vi "PathPlanner_Trajectory_CalculateMaxVel.vi"(8 "Reversed":bool, 9 "MaxAccel":dbl, 10 "MaxVel":dbl, 11 "PathPlannerStates":T1[](array[typedef]) {"HolonomicRotation"."SIN" format="%13.4f"; "HolonomicRotation"."COS" format="%13.4f"; "HolonomicRotation"."VALUE" format="%13.4f"; "AngularVelocity"."SIN" format="%13.4f"; "AngularVelocity"."COS" format="%13.4f"; "AngularVelocity"."VALUE" format="%13.4f"; "TrajectoryState"."POSE"."ROTATION"."SIN" format="%13.4f"; "TrajectoryState"."POSE"."ROTATION"."COS" format="%13.4f"; "TrajectoryState"."POSE"."ROTATION"."VALUE" format="%13.4f"; "TrajectoryState"."POSE"."TRANSLATION"."Y" format="%14.3f"; "TrajectoryState"."POSE"."TRANSLATION"."X" format="%14.3f"; "AngularAcceleration"."SIN" format="%13.4f"; "AngularAcceleration"."COS" format="%13.4f"; "AngularAcceleration"."VALUE" format="%13.4f"}) -> (3 "outPathPlannerStates":T1[](array[typedef]) {"HolonomicRotation"."SIN" format="%13.4f"; "HolonomicRotation"."COS" format="%13.4f"; "HolonomicRotation"."VALUE" format="%13.4f"; "AngularVelocity"."SIN" format="%13.4f"; "AngularVelocity"."COS" format="%13.4f"; "AngularVelocity"."VALUE" format="%13.4f"; "TrajectoryState"."POSE"."ROTATION"."SIN" format="%13.4f"; "TrajectoryState"."POSE"."ROTATION"."COS" format="%13.4f"; "TrajectoryState"."POSE"."ROTATION"."VALUE" format="%13.4f"; "TrajectoryState"."POSE"."TRANSLATION"."Y" format="%14.3f"; "TrajectoryState"."POSE"."TRANSLATION"."X" format="%14.3f"; "AngularAcceleration"."SIN" format="%13.4f"; "AngularAcceleration"."COS" format="%13.4f"; "AngularAcceleration"."VALUE" format="%13.4f"})   [LabVIEW 2019, in "PathPlanner.lvlib"]
uses:
  PathPlanner.lvlib
  PathPlannerState.ctl
  <vilib>/Rock Robotics/WPI/ThirdParty/JAS_Junk/TrajLib/ROTATION2D.ctl
  <vilib>/Rock Robotics/WPI/ThirdParty/JAS_Junk/TrajLib/TRAJ_STATE.ctl
  <vilib>/Rock Robotics/WPI/ThirdParty/JAS_Junk/TrajLib/POSE2D.ctl
  <vilib>/Rock Robotics/WPI/ThirdParty/JAS_Junk/TrajLib/TRANSLATION2D.ctl
  <vilib>/Rock Robotics/WPI/ThirdParty/JAS_Junk/TrajLib/Trajectory_Library.lvlib
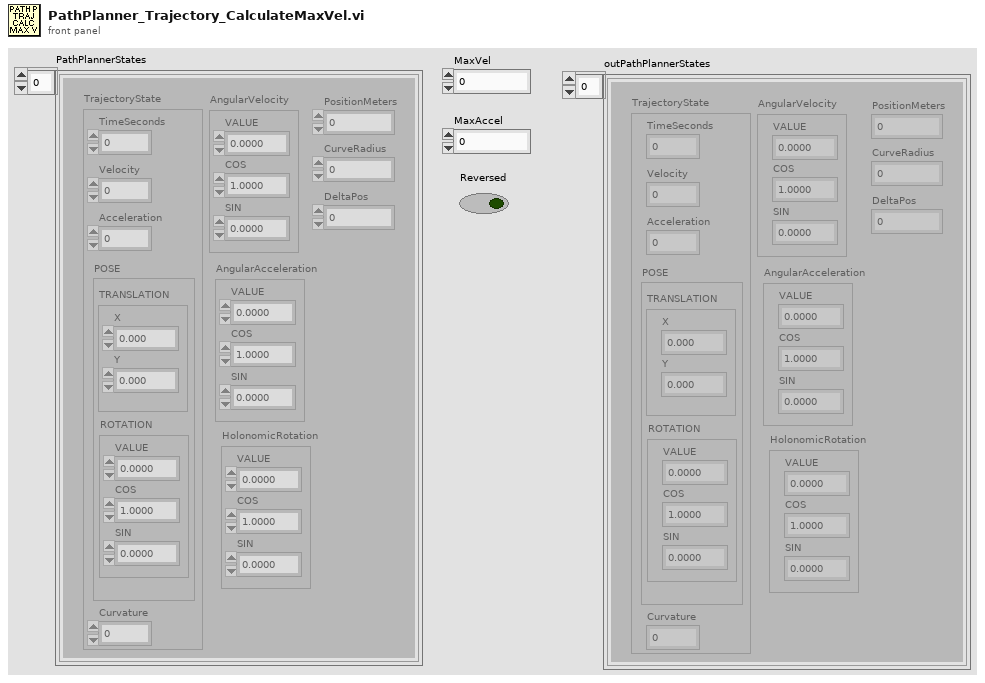
[diagram p1: front panel]
types:
  T1 = typedef "PathPlanner.lvlib/PathPlannerState.ctl" = cluster{"AngularAcceleration":T2, "PositionMeters":dbl, "TrajectoryState":T3, "AngularVelocity":T2, "HolonomicRotation":T2, "CurveRadius":dbl, "DeltaPos":dbl}
  T2 = typedef "Trajectory_Library.lvlib/ROTATION2D.ctl" = cluster{"VALUE":dbl, "COS":dbl, "SIN":dbl}
  T3 = typedef "Trajectory_Library.lvlib/TRAJ_STATE.ctl" = cluster{"TimeSeconds":dbl, "Velocity":dbl, "Acceleration":dbl, "POSE":T4, "Curvature":dbl}
  T4 = typedef "Trajectory_Library.lvlib/POSE2D.ctl" = cluster{"TRANSLATION":T5, "ROTATION":T2}
  T5 = typedef "Trajectory_Library.lvlib/TRANSLATION2D.ctl" = cluster{"X":dbl, "Y":dbl}
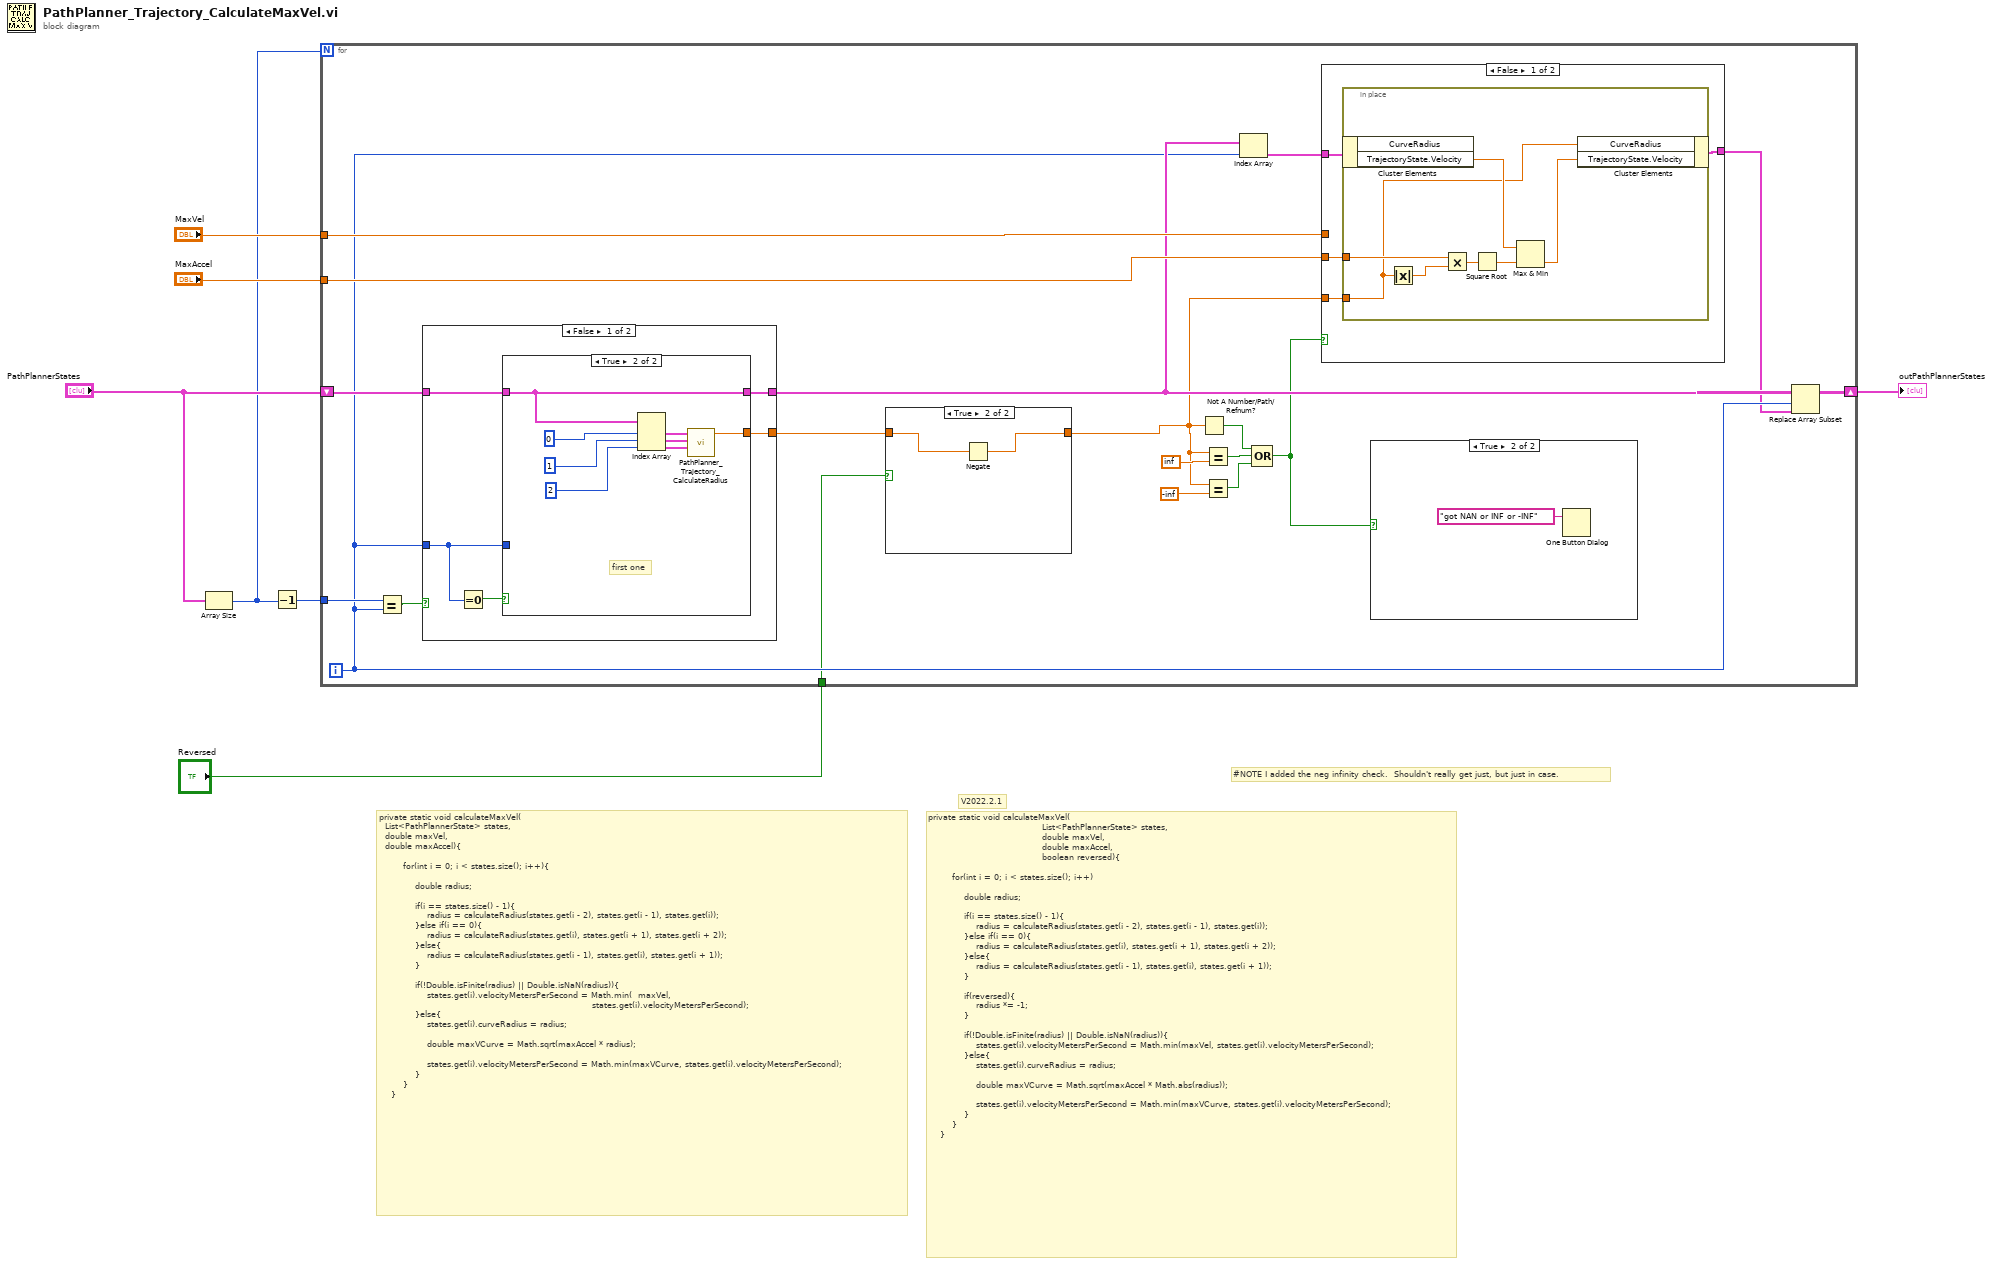
[diagram p0: block diagram]
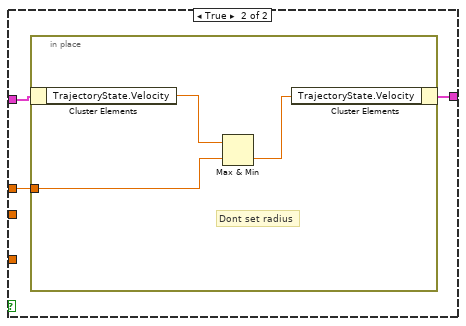
[diagram p4: hidden frame]
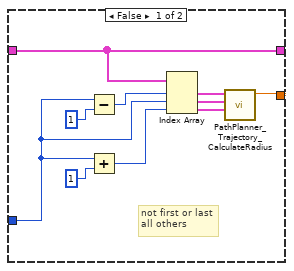
[diagram p5: hidden frame]
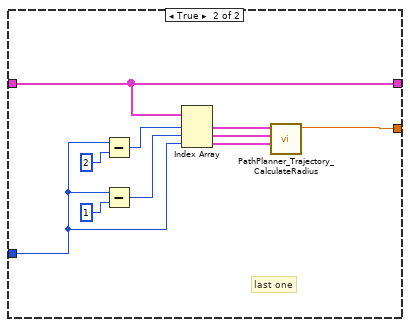
[diagram p6: hidden frame]
diagram:
  # "V2022.2.1"
  # "private static void calculateMaxVel(\n                                      List<PathPlannerState> states, \n                                      double maxVel, \n                                      double maxAccel, \n                                      boolean reversed){\n\n        for(int i = 0; i < states.size(); i++)\n\n            double radius;\n\n            if(i == states.size() - 1){\n                radius = calculateRadius(states.get(i - 2), states.get(i - 1), states.get(i));\n            }else if(i == 0){\n                radius = calculateRadius(states.get(i), states.get(i + 1), states.get(i + 2));\n            }else{\n                radius = calculateRadius(states.get(i - 1), states.get(i), states.get(i + 1));\n            }\n\n            if(reversed){\n                radius *= -1;\n            }\n\n            if(!Double.isFinite(radius) || Double.isNaN(radius)){\n                states.get(i).velocityMetersPerSecond = Math.min(maxVel, states.get(i).velocityMetersPerSecond);\n            }else{\n                states.get(i).curveRadius = radius;\n\n                double maxVCurve = Math.sqrt(maxAccel * Math.abs(radius));\n\n                states.get(i).velocityMetersPerSecond = Math.min(maxVCurve, states.get(i).velocityMetersPerSecond);\n            }\n        }\n    }"
  # "private static void calculateMaxVel(\n\t\tList<PathPlannerState> states, \n\t\tdouble maxVel, \n\t\tdouble maxAccel){\n\n        for(int i = 0; i < states.size(); i++){\n\n            double radius;\n\n            if(i == states.size() - 1){\n                radius = calculateRadius(states.get(i - 2), states.get(i - 1), states.get(i));\n            }else if(i == 0){\n                radius = calculateRadius(states.get(i), states.get(i + 1), states.get(i + 2));\n            }else{\n                radius = calculateRadius(states.get(i - 1), states.get(i), states.get(i + 1));\n            }\n\n            if(!Double.isFinite(radius) || Double.isNaN(radius)){\n                states.get(i).velocityMetersPerSecond = Math.min(  maxVel, \n\t\t\t\t                                                                   states.get(i).velocityMetersPerSecond);\n            }else{\n                states.get(i).curveRadius = radius;\n\n                double maxVCurve = Math.sqrt(maxAccel * radius);\n\n                states.get(i).velocityMetersPerSecond = Math.min(maxVCurve, states.get(i).velocityMetersPerSecond);\n            }\n        }\n    }"
  # "#NOTE I added the neg infinity check.  Shouldn't really get just, but just in case."
  n1 = Array Size(array="PathPlannerStates") -> (size(s)=w2:i32)
  n2 = Decrement(x=w2) -> (x-1=w7:i32)
  n3 = for {
    N: w2 -> [_]
    tunnel: w7 -> [w26]
    tunnel: "MaxVel" -> [w18]
    tunnel: "MaxAccel" -> [w17]
    shift-right: [w15] -> w3
    shift-left: "PathPlannerStates" -> [w24]
    tunnel: "Reversed" -> [w8]
    i -> [w13]
    n4 = Equal?(x=w26, y=w13) -> (x = y?=w25:bool)
    n5 = case shown="False" w25 {
      tunnel: w24 -> [w51 w71]
      tunnel: w13 -> [w49 w76]
      tunnel: [w50 w72] -> w10
      tunnel: [w48 w71] -> w14
      frame False {
        n6 = Equal To 0?(x=w49) -> (x = 0?=w52:bool)
        n7 = case shown="True" w52 {
          tunnel: w51 -> [w53 w63]
          tunnel: [w54 w64] -> w50
          tunnel: w49 -> [w56 _]
          tunnel: [w53 w63] -> w48
          frame False {
            # "not first or last\nall others"
            n8 = Subtract(x=w56, y=1) -> (x-y=w60:i32)
            n9 = Add(x=w56, y=1) -> (x+y=w55:i32)
            n10 = Index Array(array=w53, index #1=w60, index #2=w56, index #3=w55) -> (element #1=w59:T1, element #2=w58:T1, element #3=w57:T1)
            n11 = call "PathPlanner_Trajectory_CalculateRadius.vi"("S2"=w57, "S1"=w58, "S0"=w59) -> ("Radius"=w54:dbl)  [unwired: 8 in]
          }
          frame True {
            # "first one"
            n12 = Index Array(array=w63, index #1=0 ("y"), index #2=1 ("y"), index #3=2 ("y")) -> (element #1=w70:T1, element #2=w69:T1, element #3=w68:T1)
            n13 = call "PathPlanner_Trajectory_CalculateRadius.vi"("S2"=w68, "S1"=w69, "S0"=w70) -> ("Radius"=w64:dbl)  [unwired: 8 in]
          }
        }
      }
      frame True {
        # "last one"
        n14 = Subtract(x=w76, y=2) -> (x-y=w78:i32)
        n15 = Subtract(x=w76, y=1) -> (x-y=w77:i32)
        n16 = Index Array(array=w71, index #1=w78, index #2=w77, index #3=w76) -> (element #1=w75:T1, element #2=w74:T1, element #3=w73:T1)
        n17 = call "PathPlanner_Trajectory_CalculateRadius.vi"("S2"=w73, "S1"=w74, "S0"=w75) -> ("Radius"=w72:dbl)  [unwired: 8 in]
      }
    }
    n18 = case shown="True" w8 {
      tunnel: w10 -> [w27 w29]
      tunnel: [w27 w28] -> w9
      frame False {
      }
      frame True {
        n19 = Negate(x=w29) -> (-x=w28:dbl)
      }
    }
    n20 = Not A Number/Path/Refnum?(number/path/refnum=w9) -> (NaN/Path/Refnum?=w21:bool)
    n21 = Equal?(x=w9, y=inf) -> (x = y?=w20:bool)
    n22 = Equal?(x=w9, y=-inf) -> (x = y?=w19:bool)
    n23 = Index Array(array=w14, index=w13) -> (element=w16:T1)
    n24 = Compound Arithmetic op=OR(w21, w20, w19) -> (w11:bool)
    n25 = case shown="False" w11 {
      tunnel: [w34 w44] -> w12
      tunnel: w18 -> [_ w43]
      tunnel: w9 -> [w33 _]
      tunnel: w17 -> [w32 _]
      tunnel: w16 -> [w31 w42]
      frame False {
        n26 = in-place {
          in-place-border: w33 -> [w36]
          in-place-border: w32 -> [w41]
          n27 = in-place-cluster #1(w31) -> ("TrajectoryState.Velocity"=w37:dbl)  [unwired: 1 out]
          n28 = Absolute Value(x=w36) -> (abs(x)=w35:dbl)
          n29 = Multiply(x=w41, y=w35) -> (x*y=w40:dbl)
          n30 = Square Root(x=w40) -> (sqrt(x)=w39:dbl)
          n31 = Max & Min(x=w37, y=w39) -> (min(x,y)=w38:dbl)  [unwired: 1 out]
          n32 = in-place-cluster #1("CurveRadius"=w36, "TrajectoryState.Velocity"=w38) -> (w34:T1)
        }
      }
      frame True {
        n33 = in-place {
          in-place-border: w43 -> [w46]
          # "Dont set radius"
          n34 = in-place-cluster #2(w42) -> ("TrajectoryState.Velocity"=w45:dbl)
          n35 = Max & Min(x=w45, y=w46) -> (min(x,y)=w47:dbl)  [unwired: 1 out]
          n36 = in-place-cluster #2("TrajectoryState.Velocity"=w47) -> (w44:T1)
        }
      }
    }
    n37 = case shown="True" w11 {
      frame False {
      }
      frame True {
        n38 = One Button Dialog(message="got NAN or INF or -INF") -> ()  [unwired: 1 in, 1 out]
      }
    }
    n39 = Replace Array Subset(array=w14, new element=w12, index=w13) -> (w15:T1[])
  }
  "outPathPlannerStates" <- w3
